vi "CRYGet Graph Data in Graph.vi"(8 "sOption":string, 9 "Graph Type":string="XY", 10 "Legend Refnum":refnum<vi>, 11 "Type In":enum16{"Curves", "Values", "Results", "WFM"}(ring)) -> (0 "Result Rows":i32[](array[numeric]), 1 "Value Rows":i32[](array[numeric]), 2 "Rows":i32[](array[numeric]), 3 "Type Out":enum16{"Curves", "Values", "Results", "WFM"}(ring), 4 "Item Symbols":i32[](array[numeric]))   [LabVIEW 2013]
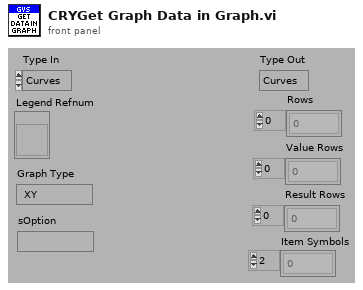
[diagram p1: front panel]
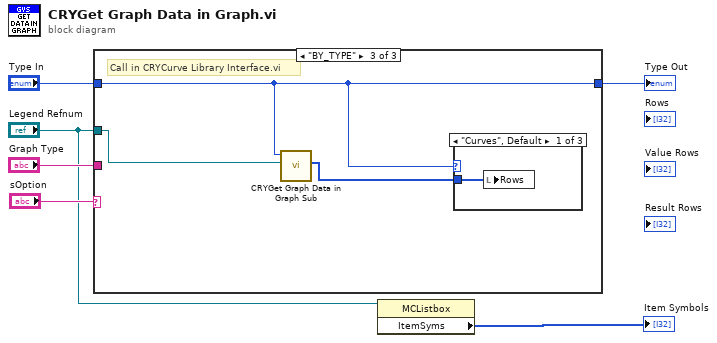
[diagram p0: block diagram]
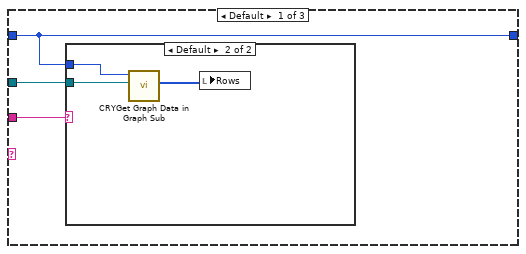
[diagram p2: hidden frame]
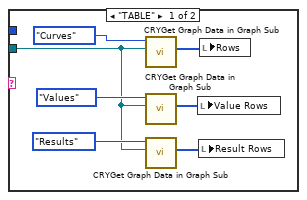
[diagram p3: hidden frame]
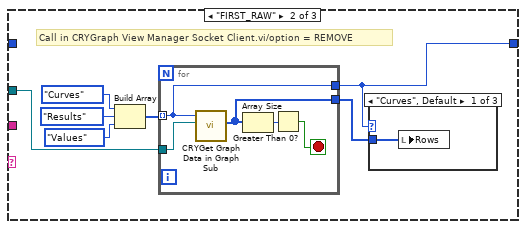
[diagram p4: hidden frame]
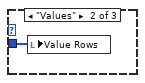
[diagram p5: hidden frame]
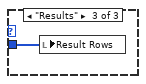
[diagram p6: hidden frame]
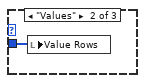
[diagram p7: hidden frame]
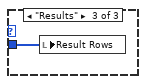
[diagram p8: hidden frame]
diagram:
  n1 = case shown="\"BY_TYPE\"" "sOption" {
    tunnel: "Type In" -> [w7 _ w35]
    tunnel: "Graph Type" -> [w9 _ _]
    tunnel: "Legend Refnum" -> [w8 w20 w36]
    tunnel: [w7 w26 w35] -> w3
    frame Default {
      n2 = case shown="Default" w9 {
        tunnel: w8 -> [w13 w18]
        tunnel: w7 -> [_ w19]
        frame "TABLE" {
          n3 = call "CRYGet Graph Data in Graph Sub.vi"("Legend Refnum"=w13, "Type In"=enum16{"Curves", "Values", "Results", "WFM"}."Curves" ("Type")) -> ("Rows"=w12:i32[])  [unwired: 5 in, 4 out]
          n4 = call "CRYGet Graph Data in Graph Sub.vi"("Legend Refnum"=w13, "Type In"=enum16{"Curves", "Values", "Results", "WFM"}."Values") -> ("Rows"=w11:i32[])  [unwired: 5 in, 4 out]
          n5 = call "CRYGet Graph Data in Graph Sub.vi"("Legend Refnum"=w13, "Type In"=enum16{"Curves", "Values", "Results", "WFM"}."Results") -> ("Rows"=w10:i32[])  [unwired: 5 in, 4 out]
          n6 = local write "Value Rows"(w11) -> ()
          n7 = local write "Result Rows"(w10) -> ()
          n8 = local write "Rows"(w12) -> ()
        }
        frame Default {
          n9 = call "CRYGet Graph Data in Graph Sub.vi"("Legend Refnum"=w18, "Type In"=w19) -> ("Rows"=w17:i32[])  [unwired: 5 in, 4 out]
          n10 = local write "Rows"(w17) -> ()
        }
      }
    }
    frame "FIRST_RAW" {
      # "Call in CRYGraph View Manager Socket Client.vi/option = REMOVE"
      n11 = Build Array(enum16{"Curves", "Values", "Results", "WFM"}."Curves" ("Type In"), enum16{"Curves", "Values", "Results", "WFM"}."Results" ("Type In"), enum16{"Curves", "Values", "Results", "WFM"}."Values" ("Type In")) -> (w24:enum16{"Curves", "Values", "Results", "WFM"}[])
      n12 = for {
        tunnel: w24 -> [w29] mode=indexing
        tunnel: [w29] -> w26
        tunnel: [w28] -> w25
        tunnel: w20 -> [w27]
        stop <- w30 stop-if-true
        n13 = call "CRYGet Graph Data in Graph Sub.vi"("Legend Refnum"=w27, "Type In"=w29) -> ("Rows"=w28:i32[])  [unwired: 5 in, 4 out]
        n14 = Array Size(array=w28) -> (size(s)=w31:i32)
        n15 = Greater Than 0?(x=w31) -> (x > 0?=w30:bool)
      }
      n16 = case shown="\"Curves\", Default" w26 {
        tunnel: w25 -> [w32 w33 w34]
        frame "Curves", Default {
          n17 = local write "Rows"(w32) -> ()
        }
        frame "Values" {
          n18 = local write "Value Rows"(w33) -> ()
        }
        frame "Results" {
          n19 = local write "Result Rows"(w34) -> ()
        }
      }
    }
    frame "BY_TYPE" {
      # "Call in CRYCurve Library Interface.vi"
      n20 = call "CRYGet Graph Data in Graph Sub.vi"("Legend Refnum"=w36, "Type In"=w35) -> ("Rows"=w37:i32[])  [unwired: 5 in, 4 out]
      n21 = case shown="\"Curves\", Default" w35 {
        tunnel: w37 -> [w38 w39 w40]
        frame "Curves", Default {
          n22 = local write "Rows"(w38) -> ()
        }
        frame "Values" {
          n23 = local write "Value Rows"(w39) -> ()
        }
        frame "Results" {
          n24 = local write "Result Rows"(w40) -> ()
        }
      }
    }
  }
  "Type Out" <- w3
  n25 = property class="MCListbox"(reference="Legend Refnum") -> ("ItemSyms"=→"Item Symbols":i32[])  [unwired: 1 in, 2 out]
